vi "2.2.vi"() -> ()   [LabVIEW 2020]
uses:
  <vilib>/numeric/Random Number (Range) I64.vi
  <vilib>/numeric/sub_Random U32.vi
panel:
  out "Minimo":dbl
  out "Maximo":dbl
  out "temperaturas":dbl[][](array[numeric])
  # "fahrenheit"
  # "celsius"
  # "ema"
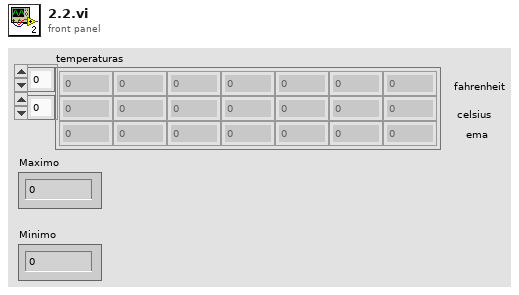
[diagram p1: front panel]
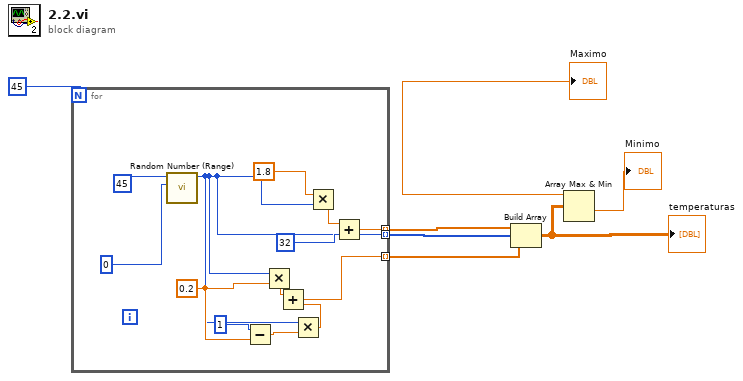
[diagram p0: block diagram]
diagram:
  n1 = for {
    N: 45 -> [_]
    tunnel: [w15] -> w6 mode=indexing
    tunnel: [w8] -> w5 mode=indexing
    tunnel: [w9] -> w4 mode=indexing
    w13 = 0.2
    n2 = call-poly <vilib>:"Random Number (Range).vi"("lower bound (-100)"=0, "upper bound (100)"=45) -> ("number"=w8:i64)  [unwired: 9 in]
    n3 = Subtract(x=1, y=w13) -> (x-y=w10:dbl)
    n4 = Multiply(x=w8, y=w13) -> (x*y=w12:dbl)
    n5 = Multiply(x=w8, y=w10) -> (x*y=w11:dbl)
    n6 = Add(x=w12, y=w11) -> (x+y=w9:dbl)
    n7 = Multiply(x=1.8, y=w8) -> (x*y=w17:dbl)
    n8 = Add(x=w17, y=32) -> (x+y=w15:dbl)
  }
  n9 = Build Array(w6, w5, w4) -> (w3:dbl[][])
  "temperaturas" <- w3
  n10 = Array Max & Min(array=w3) -> (max value=→"Maximo":dbl, min value=→"Minimo":dbl)  [unwired: 2 out]
